vi "stateExecution.vi"(8 "error in (no error)":errorcluster, 11 "statemachine in":refnum<class "statemachine.lvclass">) -> (0 "error out":errorcluster, 3 "statemachine out":refnum<class "statemachine.lvclass">)   [LabVIEW 2020, in "eos.lvlib" / "statemachine.lvclass"]
uses:
  statemachine.lvclass
  interfaces/state/state.lvclass
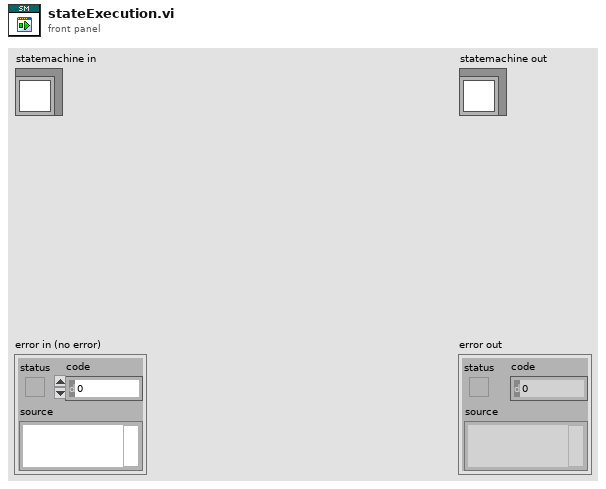
[diagram p1: front panel]
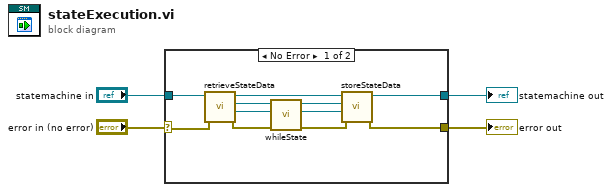
[diagram p0: block diagram]
diagram:
  n1 = case shown="No Error" "error in (no error)" {
    selector: "error in (no error)" -> [w8 w16]
    tunnel: [w6 w16] -> w3
    tunnel: [w5 w17] -> w2
    tunnel: "statemachine in" -> [w15 w17]
    frame No Error {
      n2 = call "retrieveStateData.vi"("error in (no error)"=w8, "statemachine in"=w15) -> ("error out"=w9:errorcluster, "State Data"=w11:refnum<class "data.lvclass">, "State"=w13:refnum<class "state.lvclass">, "statemachine out"=w14:refnum<class "statemachine.lvclass">)  [unwired: 6 in]
      n3 = call-dynamic "whileState.vi"("error in (no error)"=w9, "State Data in"=w11, "state in"=w13) -> ("error out"=w7:errorcluster, "State Data out"=w10:refnum<class "data.lvclass">, "state out"=w12:refnum<class "state.lvclass">)  [unwired: 6 in]
      n4 = call "storeStateData.vi"("error in (no error)"=w7, "State Data"=w10, "Current State"=w12, "statemachine in"=w14) -> ("error out"=w6:errorcluster, "statemachine out"=w5:refnum<class "statemachine.lvclass">)  [unwired: 5 in, 1 out]
    }
    frame Error {
    }
  }
  "error out" <- w3
  "statemachine out" <- w2
